vi "Initial, set and read, loop, pause (20220808).vi"() -> ()   [LabVIEW 2017]
panel:
  out "Scan Times":i32
  in  "stop":bool
  out "Paused":bool
  in  "Pause Request":bool
  out "Message":string
  in  "Mono Wait time (ms)":u32=5000
  out "Wavelength Set":bool
  out "Total points":i32=5
  out "WL Range":dbl[](array[numeric])=[800.0, 850.0, 900.0, 950.0, 1000.0]
  in  "Step size (nm)":sgl=50.0 min=1 step=0.1
  in  "End Wavelength (nm)":dbl=1300.0 min=250.0 max=1350.0 step=0.1
  in  "Start Wavelength (nm)":dbl=500.0 min=250.0 max=1200.0 step=0.1
  out "Current wavelength":dbl=900.0
  out "Mono status":bool
  out "Output Wavelength":dbl=849.997 min=350.0 max=1100.0 step=1.0 format="%#.1f"
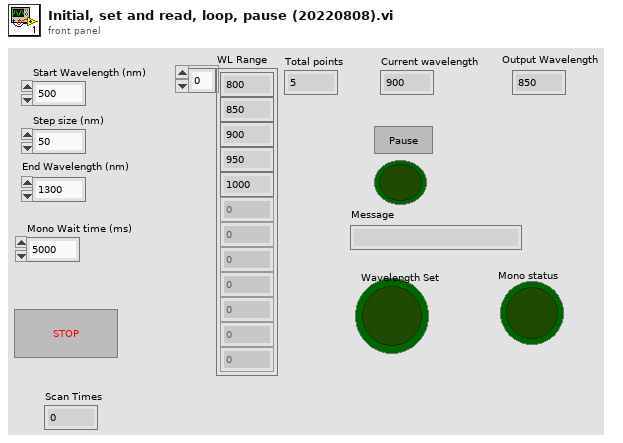
[diagram p1: front panel]
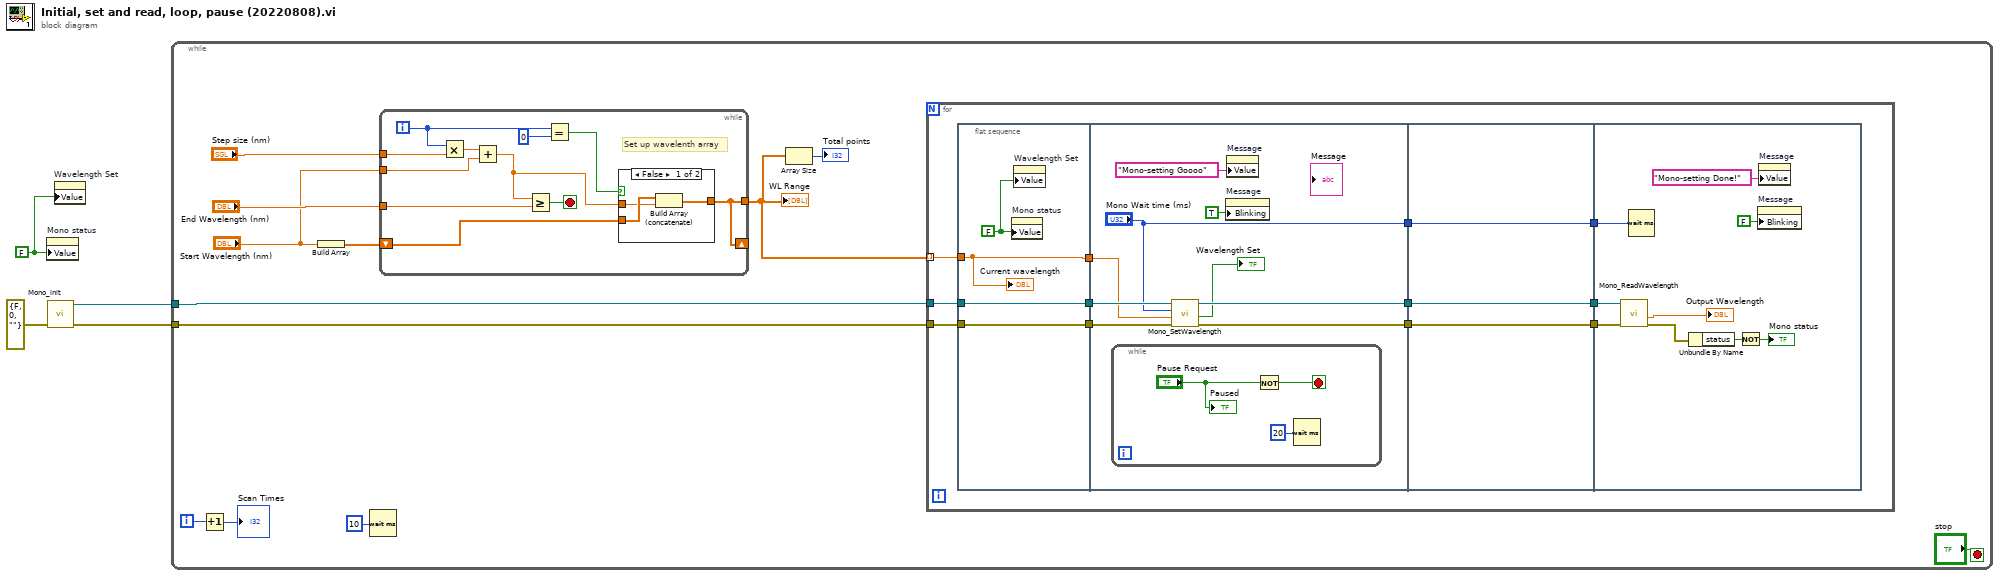
[diagram p0: block diagram]
diagram:
  w4 = FALSE ("Mono status")
  n1 = property on="Mono status" class="Bool (strict)"("Value"=w4) -> ()  [unwired: 2 in, 2 out]
  n2 = call "Mono_init.vi"("error in (no error)"=errorcluster {"status"=FALSE, "code"=0, "source"=""}) -> ("error out"=w1:errorcluster, "CmdLib"=w2:refnum<k24>)  [unwired: 8 in, 1 out]
  n3 = property on="Wavelength Set" class="Bool (strict)"("Value"=w4) -> ()  [unwired: 2 in, 2 out]
  n4 = while {
    tunnel: w2 -> [w15]
    tunnel: w1 -> [w14]
    i -> [w6]
    stop <- "stop" stop-if-true
    n5 = Increment(x=w6) -> (x+1=→"Scan Times":i32)
    n6 = Build Array "Build Array"("Start Wavelength (nm)") -> (w10:dbl[])
    n7 = Wait (ms)(milliseconds to wait=u32 10) -> ()  [unwired: 1 out]
    n8 = while {
      shift-right: [w57] -> _
      shift-left: w10 -> [w59]
      tunnel: "Step size (nm)" -> [w66]
      tunnel: "End Wavelength (nm)" -> [w67]
      tunnel: "Start Wavelength (nm)" -> [w60]
      tunnel: [w57] -> w16
      i -> [w62]
      stop <- w64 stop-if-true
      # "Set up wavelenth array"
      n9 = Multiply(x=w62, y=w66) -> (x*y=w65:sgl)
      n10 = Add(x=w65, y=w60) -> (x+y=w58:dbl)
      n11 = Greater Or Equal?(x=w58, y=w67) -> (x >= y?=w64:bool)
      n12 = Equal?(x=w62, y=0) -> (x = y?=w61:bool)
      n13 = case shown="False" w61 {
        tunnel: w59 -> [w70 w71]
        tunnel: w58 -> [w69 _]
        tunnel: [w68 w71] -> w57
        frame False {
          n14 = Build Array (concatenate)(w70, w69) -> (w68:dbl[])
        }
        frame True {
        }
      }
    }
    "WL Range" <- w16
    n15 = Array Size(array=w16) -> (size(s)=→"Total points":i32)
    n16 = for {
      tunnel: w14 -> [w26]
      tunnel: w15 -> [w27]
      tunnel: w16 -> [w28] mode=indexing
      n17 = flat-sequence {
        tunnel: w28 -> [w32]
        tunnel: w27 -> [w31]
        tunnel: w26 -> [w30]
        tunnel: [w32] -> w25
        tunnel: [w31] -> w24
        tunnel: [w30] -> w23
        tunnel: w25 -> [w39]
        tunnel: w24 -> [w40]
        tunnel: w23 -> [w41]
        tunnel: [w38] -> w20
        tunnel: [w37] -> w22
        tunnel: ["Mono Wait time (ms)"] -> w18
        tunnel: w22 -> [w47]
        tunnel: [w47] -> w21
        tunnel: w20 -> [w46]
        tunnel: [w46] -> w19
        tunnel: w18 -> [w45]
        tunnel: [w45] -> w17
        tunnel: w21 -> [w51]
        tunnel: w19 -> [w52]
        tunnel: w17 -> [w49]
        frame #0 {
          w29 = FALSE ("Mono status")
          n18 = property on="Mono status" class="Bool (strict)"("Value"=w29) -> ()  [unwired: 2 in, 2 out]
          n19 = property on="Wavelength Set" class="Bool (strict)"("Value"=w29) -> ()  [unwired: 2 in, 2 out]
          "Current wavelength" <- w32
        }
        frame #1 {
          n20 = while {
            stop <- w43 stop-if-true
            n21 = Not(x="Pause Request") -> (.not. x?=w43:bool)
            n22 = Wait (ms)(milliseconds to wait=u32 20) -> ()  [unwired: 1 out]
            "Paused" <- "Pause Request"
          }
          n23 = call "Mono_SetWavelength.vi"("error in (no error) 2"=w41, "Wavelength"=w39, "Mono Wait time (ms)"="Mono Wait time (ms)", "CmdLib In"=w40) -> ("error out 2"=w38:errorcluster, "Wavelength Set"=→"Wavelength Set":bool, "CmdLib Out"=w37:refnum<k24>)  [unwired: 5 in]
          n24 = property on="Message" class="Str"("Blinking"=TRUE) -> ()  [unwired: 2 in, 2 out]
          n25 = property on="Message" class="Str"("Value"="Mono-setting Goooo" ("Message")) -> ()  [unwired: 2 in, 2 out]
        }
        frame #2 {
        }
        frame #3 {
          n26 = call "Mono_ReadWavelength.vi"("error in (no error) 2"=w52, "CmdLib In"=w51) -> ("error out 2"=w53:errorcluster, "getWavelength"=→"Output Wavelength":dbl)  [unwired: 7 in, 1 out]
          n27 = Wait (ms)(milliseconds to wait=w49) -> ()  [unwired: 1 out]
          n28 = Unbundle By Name(w53) -> ("status"=w55:bool)
          n29 = Not(x=w55) -> (.not. x?=→"Mono status":bool)
          n30 = property on="Message" class="Str"("Blinking"=FALSE) -> ()  [unwired: 2 in, 2 out]
          n31 = property on="Message" class="Str"("Value"="Mono-setting Done!" ("Message")) -> ()  [unwired: 2 in, 2 out]
        }
      }
    }
  }
